vi "Prefilter.60Hz_Notch.vi"(8 "error in (no error)":errorcluster, 10 "signal in":waveform(dbl)[](array[waveform]), 11 "DSP in":refnum<class "DSP.lvclass">) -> (0 "error out":errorcluster, 2 "signal out":waveform(dbl)[](array[waveform]), 3 "DSP out":refnum<class "DSP.lvclass">)   [LabVIEW 2019, in "DSP.lvclass"]
uses:
  DSP.lvclass
  DSP.lvclass/DSP.ctl
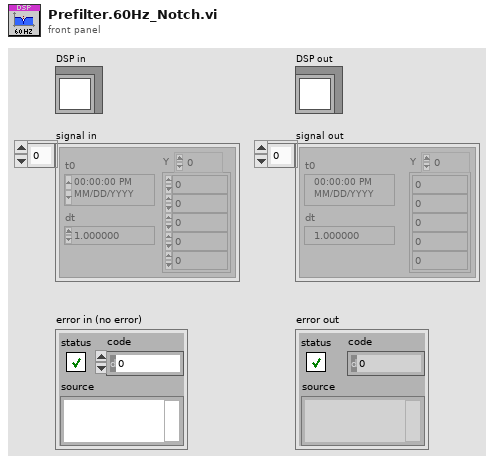
[diagram p1: front panel]
types:
  T1 = cluster{"filter structure":enum32{"IIR 2nd Order", "IIR 4th Order"}, "Reverse Coefficients":dbl[], "Forward Coefficients":dbl[]}[]
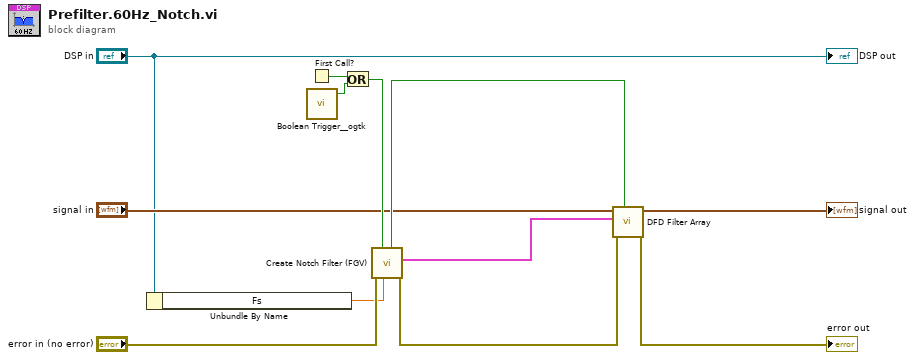
[diagram p0: block diagram]
diagram:
  n1 = Unbundle By Name("DSP in") -> ("Fs"=w1:dbl)
  n2 = First Call?() -> (First Call?: T/F=w10:bool)
  n3 = call <userlib>:"Boolean Trigger__ogtk.vi"() -> ("Rising Edge"=w8:bool)  [unwired: 2 in, 1 out]
  n4 = Or(x=w10, y=w8) -> (x .or. y?=w9:bool)
  n5 = call "Create Notch Filter (FGV).vi"("fs (Hz)"=w1, "init [F]"=w9, "error in (no error)"="error in (no error)") -> ("error out"=w5:errorcluster, "IIR Filters"=w7:T1, "init?"=w6:bool)  [unwired: 6 in]
  n6 = call "DFD Filter Array.vi"("init (F)"=w6, "error in (no error)"=w5, "IIR Filters"=w7, "signal in"="signal in") -> ("error out"=→"error out":errorcluster, "signal out"=→"signal out":waveform(dbl)[])  [unwired: 6 in]
  "DSP out" <- "DSP in"
